vi "Start BuildWorker.vi"(8 "error in (no error)":errorcluster, 9 "Show":bool=TRUE, 10 "Port":i32=4545, 11 "BuildWorker Controller in":refnum<class "BuildWorker Controller.lvclass">) -> (0 "error out":errorcluster, 3 "BuildWorker Controller out":refnum<class "BuildWorker Controller.lvclass">)   [LabVIEW 2017, in "BuildWorker Controller.lvlib" / "BuildWorker Controller.lvclass"]
uses:
  BuildWorker Controller.lvclass
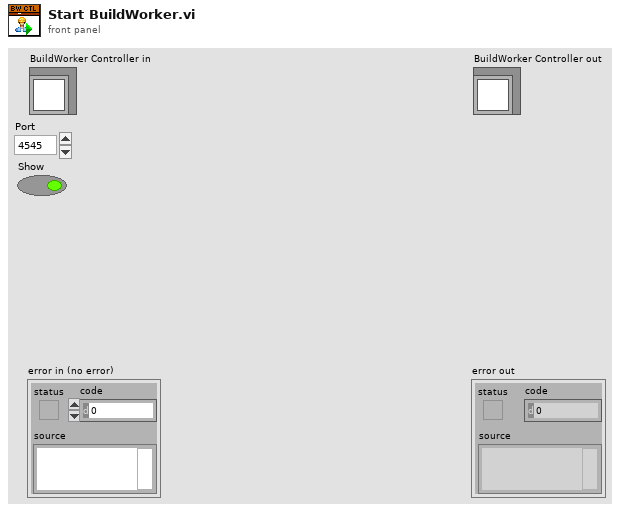
[diagram p1: front panel]
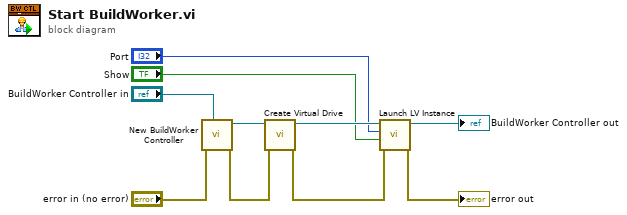
[diagram p0: block diagram]
diagram:
  n1 = call "New BuildWorker Controller.vi"("BuildWorker Controller in"="BuildWorker Controller in", "error in (no error)"="error in (no error)") -> ("error out"=w8:errorcluster, "BuildWorker Controller out"=w10:refnum<class "BuildWorker Controller.lvclass">)  [unwired: 8 in]
  n2 = call "Create Virtual Drive.vi"("error in (no error)"=w8, "BuildWorker Controller in"=w10) -> ("error out"=w7:errorcluster, "BuildWorker Controller out"=w9:refnum<class "BuildWorker Controller.lvclass">)  [unwired: 8 in]
  n3 = call "Launch LV Instance.vi"("error in (no error)"=w7, "Show"="Show", "Port"="Port", "BuildWorker Controller in"=w9) -> ("error out"=→"error out":errorcluster, "BuildWorker Controller out"=→"BuildWorker Controller out":refnum<class "BuildWorker Controller.lvclass">)  [unwired: 6 in]
